vi "NPSV test.vi"() -> ()   [LabVIEW 2019]
uses:
  DataDef.ctl
  <vilib>/NI/Modbus Library/API/Modbus API.lvclass
  <vilib>/WPC Systems Ltd/GECO Driver/Lib/GECOBase/GECO_Driver Class/GECO_Driver.lvclass
  <vilib>/WPC Systems Ltd/GECO Driver/Lib/GECOMotion/GECOMotion/_typedefine/Axis Select.ctl
  <vilib>/WPC Systems Ltd/GECO Driver/Lib/GECOBase/GECO_Driver Class/Motion/_typedefine/GECO_Stepper Output Configuration.ctl
  <vilib>/WPC Systems Ltd/GECO Driver/Lib/GECOBase/GECO_Driver Class/Motion/_typedefine/GECO_Motion Operation Mode.ctl
  <vilib>/WPC Systems Ltd/GECO Driver/Lib/GECOBase/GECO_Driver Class/GECO_SlotName.ctl
  <vilib>/WPC Systems Ltd/GECO Driver/Lib/GECOBase/GECO_Driver Class/Motion/_typedefine/GECO_ActiveHighLow.ctl
  <vilib>/WPC Systems Ltd/GECO Driver/Lib/GECOMotion/GECOMotion/GECO Motion.lvclass
  GyroDef.ctl
  <vilib>/Platform/TimedLoop/XDataNode/timing_clust.ctl
  <vilib>/Platform/TimedLoop/XDataNode/nitl_modes.ctl
  <vilib>/Platform/TimedLoop/XDataNode/wakeup.ctl
  <vilib>/NI/Modbus Library/API/Slave/Modbus Slave.lvclass
  C:/Program Files (x86)/National Instruments/LabVIEW 2019/vi.lib/NI/Modbus Library/API/Modbus API.lvclass
  <vilib>/addons/control/pid/pid.llb/PID (DBL).vi
  <vilib>/NI/Modbus Library/API/Wrapper/Create TCP Slave.vi
  <vilib>/WPC Systems Ltd/GECO Driver/GECODriver/GECO_Initialize_RT/Initialize VIs/Initialize_GECOUnoRT_4HX.vi
  <vilib>/platform/TimedLoop/XDataNode/XDataNode.xnode
  <vilib>/addons/control/pid/NI_PID_pid.lvlib
  <vilib>/NI/Modbus Library/API/Wrapper/API Main.lvlib
  <vilib>/Platform/TimedLoop/XDataNode/XDNodeRunTimeDep.lvlib
panel:
  out "error out":errorcluster
  out "Axis 1":T1
  out "Axis 2":T1
  out "Axis 3":T1
  out "Program Period":u32
  in  "Main Setting Tab":T2(tab)
  in  "PID gains setting Tab":enum32{"Axis 1", "Axis 2", "Axis 3"}(tab)
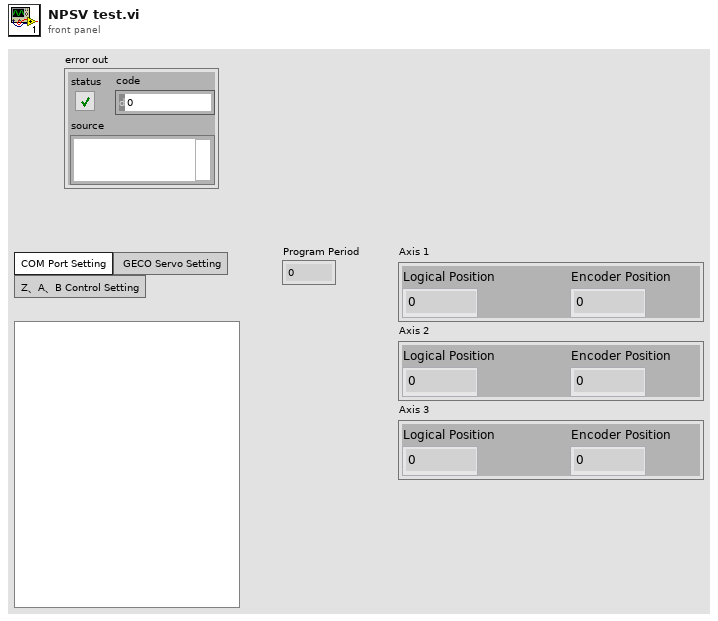
[diagram p1: front panel]
types:
  T1 = cluster{"Encoder Position":i32, "Logical Position":i32}
  T2 = enum32{"COM Port Setting", " GECO Servo Setting", "Z、A、B Control Setting"}
  T3 = typedef "DataDef.ctl" = cluster{"address starting":u16, "狀態":enum16{"初始化", "讀取", "寫入", "停止"}, "理想角度":cluster{"A":dbl, "B":dbl}, "register values":i16[], "Modbus COM":refnum<class "Modbus API.lvclass">, "TCP slave port":u16, " baud rate":u32, "Byte bits":u16, "ServoButtonControl":cluster{"三軸同退":bool, "三軸同進":bool, "三軸後退":bool, "三軸前進":bool, "二軸後退":bool, "二軸前進":bool, "一軸後退":bool, "一軸前進":bool}, "Serial Number":string, "GECO_Driver out":refnum<class "GECO_Driver.lvclass">, "number of inputs":u16, "ServoSetting":cluster{"Axis Select":T4, "Stepper Output Configuration":T5, "Motion Operation Mode":T6, "Motion Controller Slot":T7, "Singel Axis Move Paramters":cluster{"Motion Operation Mode":T6, "Target Position (0)":i32, "Velocity (10000)":i32, "Acceleration (100000)":u32, "Deacceleration (100000)":u32}, "Reverse":cluster{"Reverse Enable":bool, "Reverse Polarity":T8}, "Forward":cluster{"Forward Enable":bool, "Forward Polarity":T8}}, "GECO Motion out":refnum<class "GECO Motion.lvclass">, "Servo on":bool, "Axis 1 Position":cluster{"Encoder Position":i32, "Logical Position":i32}, "Axis 2 Position":cluster{"Encoder Position":i32, "Logical Position":i32}, "Axis 3 Position":cluster{"Encoder Position":i32, "Logical Position":i32}, "PIDSetting":cluster{"Z":i32, "A":i32, "B":i32, "Move Setting":T9, "Axis Pulse":dbl, "Axis Length":dbl, "PID gains ":cluster{"proportional gain (Kc)":dbl, "integral time (Ti, min)":dbl, "derivative time (Td, min)":dbl}}, "resource name":tag, "Save Path":refnum<file>}
  T4 = typedef "GECO Motion.lvclass/Axis Select.ctl" = enum16{"Axis 1", "Axis 2", "Axis 3", "Axis 4"}
  T5 = typedef "GECO_Driver.lvclass/GECO_Stepper Output Configuration.ctl" = enum16{"Step/Dir(One Pulse)", "CW/CCW(Two Pulse)"}
  T6 = typedef "GECO_Driver.lvclass/GECO_Motion Operation Mode.ctl" = enum16{"Absolute Position", "Relative Position", "Velocity"}
  T7 = typedef "GECO_Driver.lvclass/GECO_SlotName.ctl" = enum16{"C1", "C2", "C3", "C4"}
  T8 = typedef "GECO_Driver.lvclass/GECO_ActiveHighLow.ctl" = enum16{"Active High", "Active Low"}
  T9 = typedef "­y¸ñ.ctl" = u16
  T10 = typedef "GyroDef.ctl" = cluster{"Byte bits":u16, "baud rate":u32, "實際角度":cluster{"A":dbl, "B":dbl}, "COM Port":refnum<visa-resource-name>, "Save Path":refnum<file>}
  T11 = typedef "XDNodeRunTimeDep.lvlib/timing_clust.ctl" = cluster{"Expected End [f-1]":u64, "Actual End [f-1]":u64, "Finished Late? [f-1]":bool, "Expected End [i-1]":u64, "Actual End [i-1]":u64, "Finished Late? [i-1]":bool, "Expected Start [i]":u64, "Actual Start [i]":u64, "Expected Start [f]":u64, "Actual Start [f]":u64, "Source Name":string, "Structure Name":string, "Period":i64, "Deadline":i64, "Offset":i64, "Start":i64, "Priority":i32, "Timeout":i32, "Mode":T12, "Wakeup Reason":T13, "Error":errorcluster, "Source Type":string, "Secondary Source Type":string, "Global End Time":u64, "Global Start Time":u64, "Frame Duration":u64, "Iteration Duration":u64, "Assigned CPU":i32, "I/O Scan Engine Mode":u32}
  T12 = typedef "XDNodeRunTimeDep.lvlib/nitl_modes.ctl" = enum32{"No Change", "Process missed periods, maintain original phase", "Discard missed periods, maintain original phase", "Process missed periods, ignore original phase", "Discard missed periods, ignore original phase"}
  T13 = typedef "XDNodeRunTimeDep.lvlib/wakeup.ctl" = enum32{"Normal", "Aborted", "Asynchronous wakeup", "Timing source error", "Timed loop error", "Timeout"}
  T14 = cluster{"Motion Operation Mode":T6, "Target Position (0)":i32, "Velocity (10000)":i32, "Acceleration (100000)":u32, "Deacceleration (100000)":u32}
  T15 = cluster{"Forward Enable":bool, "Forward Polarity":T8}
  T16 = cluster{"Reverse Enable":bool, "Reverse Polarity":T8}
  T17 = cluster{"三軸同退":bool, "三軸同進":bool, "三軸後退":bool, "三軸前進":bool, "二軸後退":bool, "二軸前進":bool, "一軸後退":bool, "一軸前進":bool, "Reset Encoder Position":bool, "AlarmReset":bool}[]
  T18 = cluster{"三軸同退":bool, "三軸同進":bool, "三軸後退":bool, "三軸前進":bool, "二軸後退":bool, "二軸前進":bool, "一軸後退":bool, "一軸前進":bool, "Reset Encoder Position":bool, "AlarmReset":bool}
  T19 = enum16{"open", "replace", "create", "open or create", "replace or create", "replace or create with confirmation"}
  T20 = cluster{"Logical Position":i32, "Encoder Position":i32}
  T21 = enum16{"Step/Dir(One Pulse)", "CW/CCW(Two Pulse)"}
  T22 = enum16{"Absolute Position", "Relative Position", "Velocity"}
  T23 = cluster{"proportional gain (Kc)":dbl, "integral time (Ti, min)":dbl, "derivative time (Td, min)":dbl}
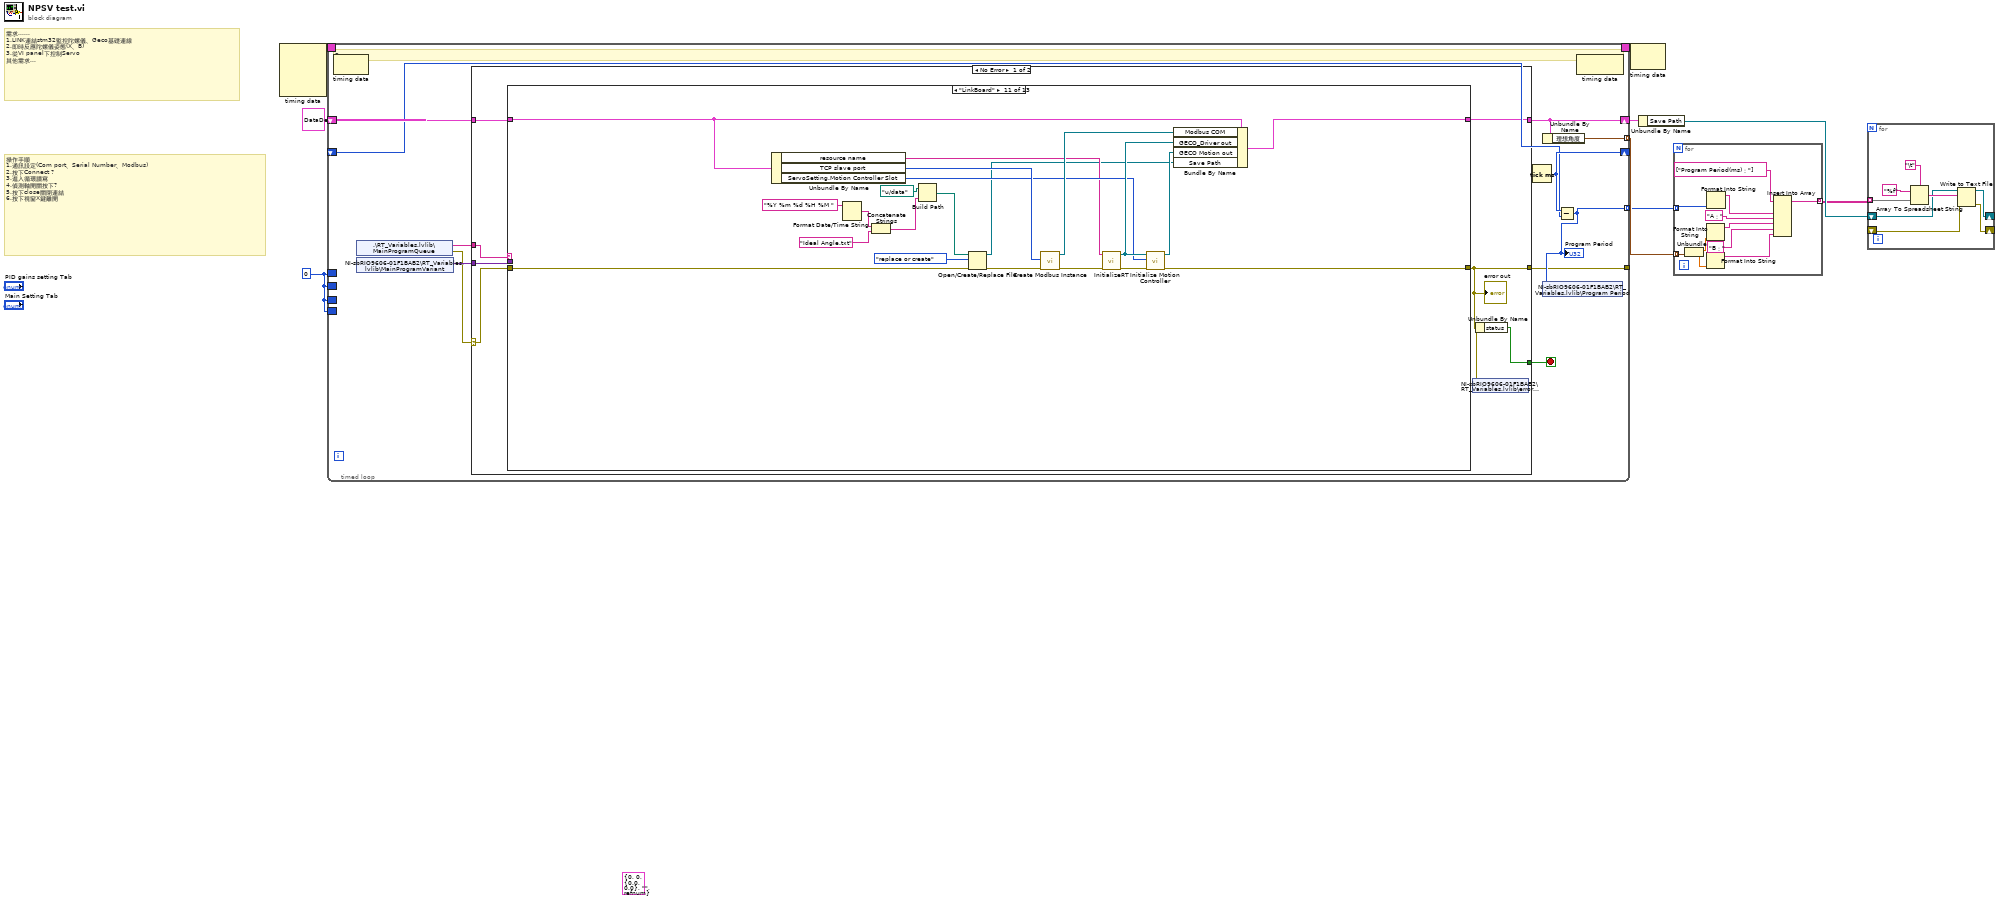
[diagram p0: block diagram]
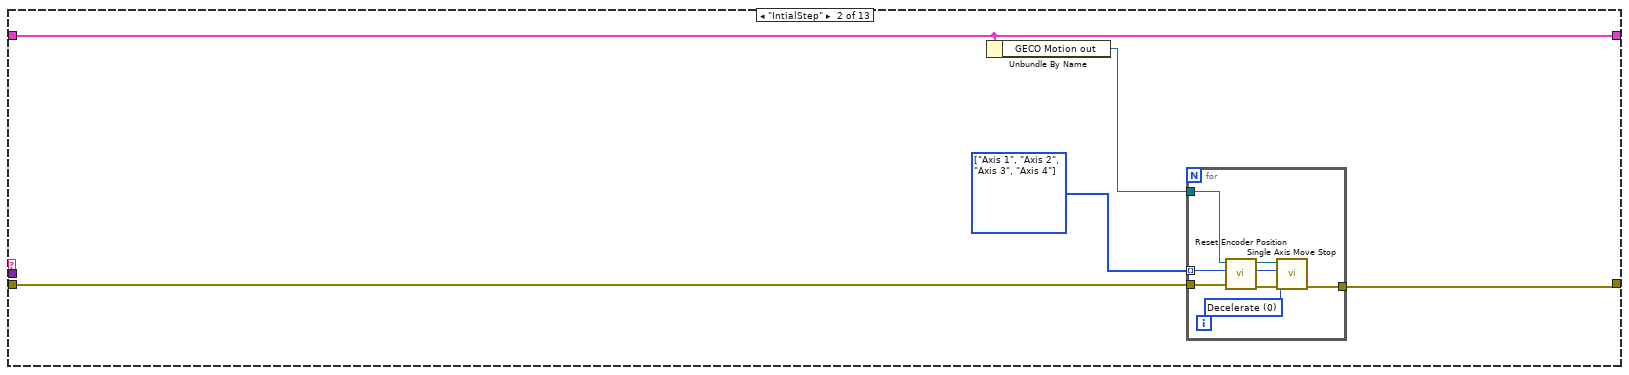
[diagram p3: hidden frame]
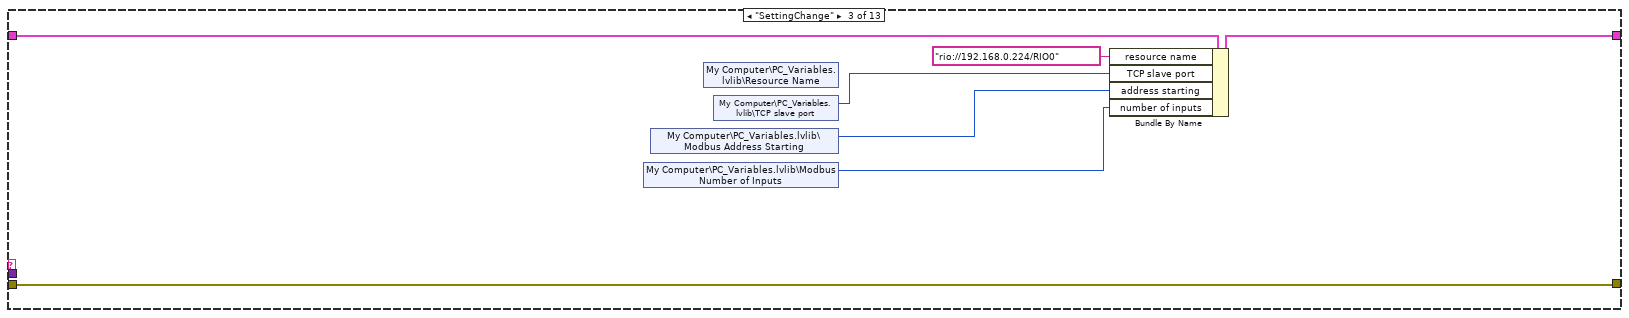
[diagram p4: hidden frame]
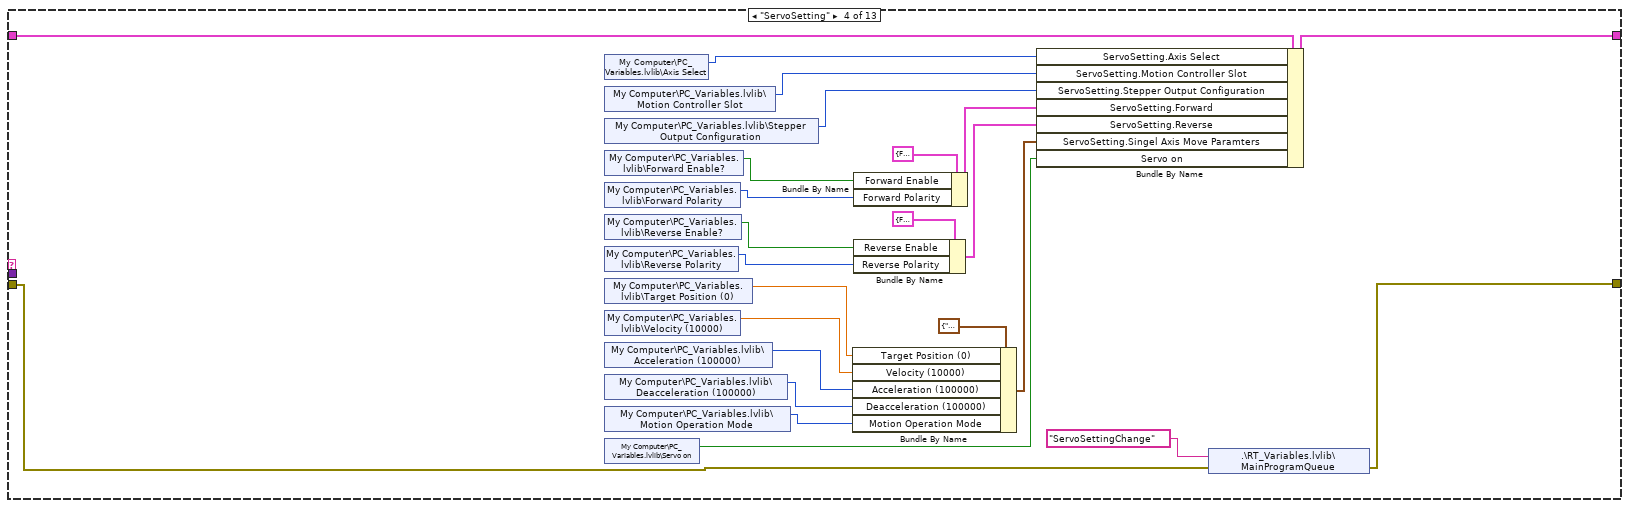
[diagram p5: hidden frame]
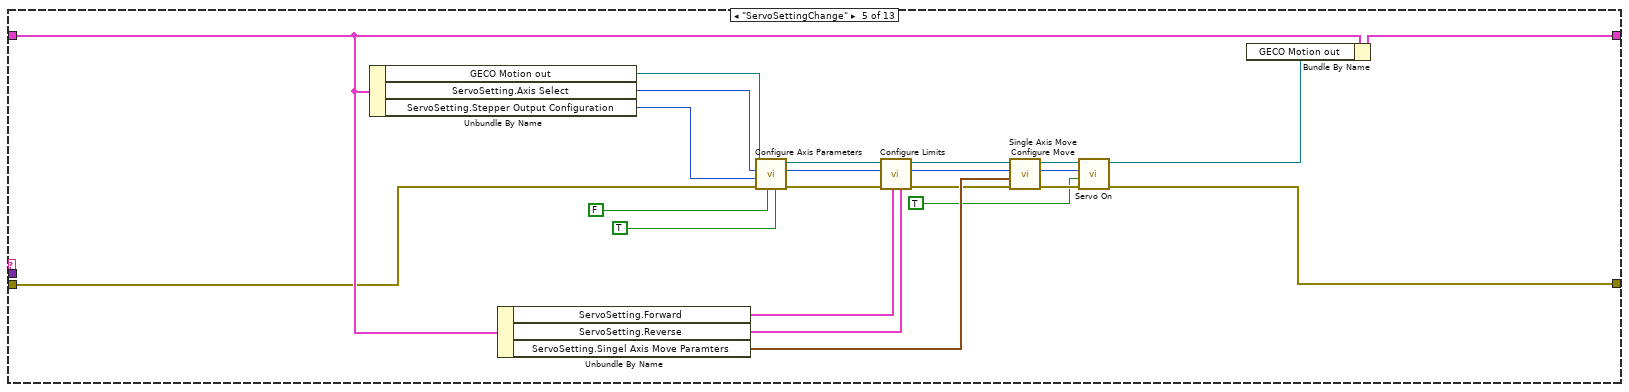
[diagram p6: hidden frame]
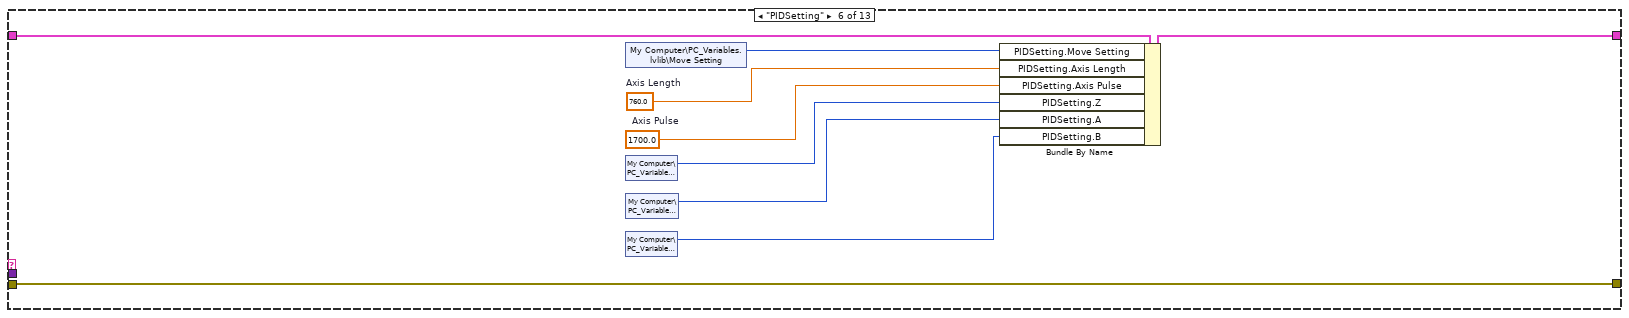
[diagram p7: hidden frame]
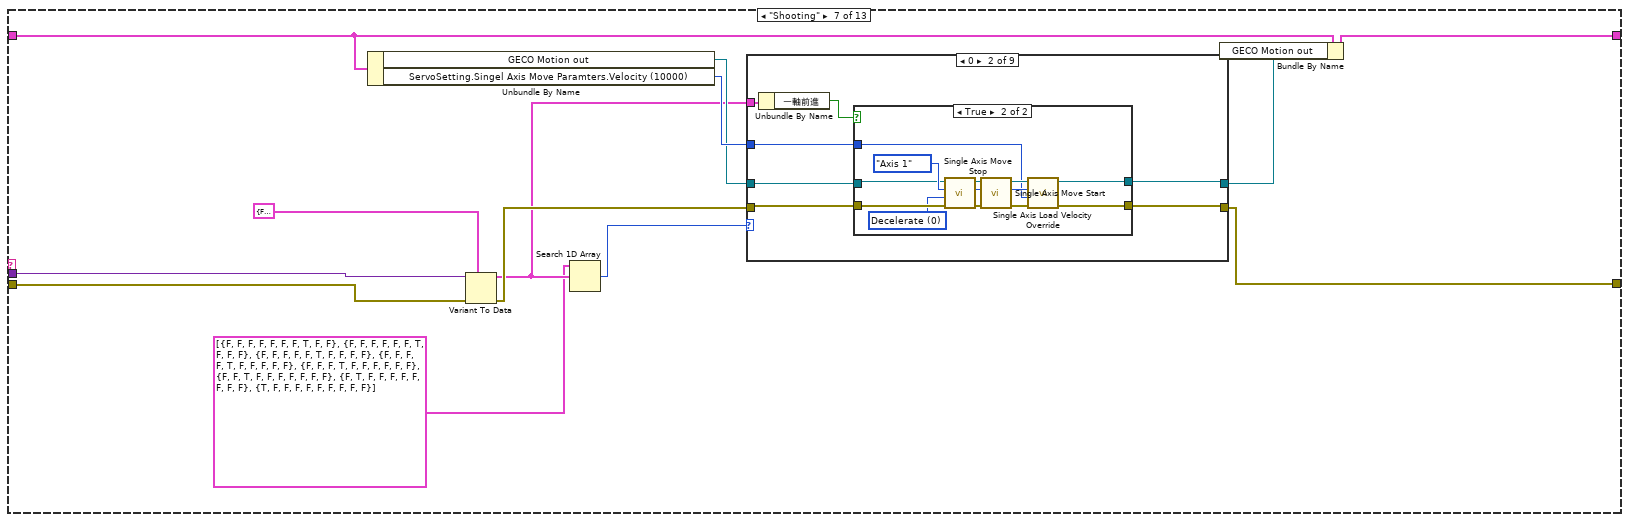
[diagram p8: hidden frame]
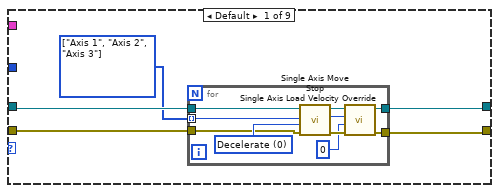
[diagram p9: hidden frame]
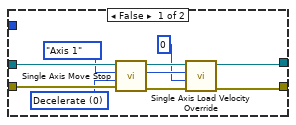
[diagram p10: hidden frame]
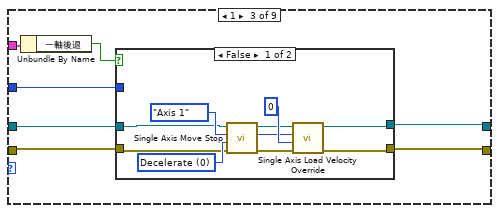
[diagram p11: hidden frame]
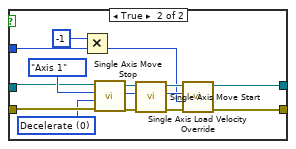
[diagram p12: hidden frame]
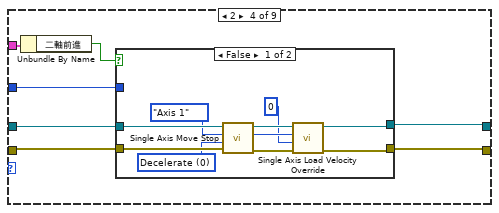
[diagram p13: hidden frame]
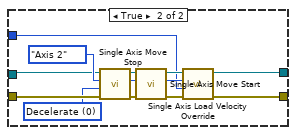
[diagram p14: hidden frame]
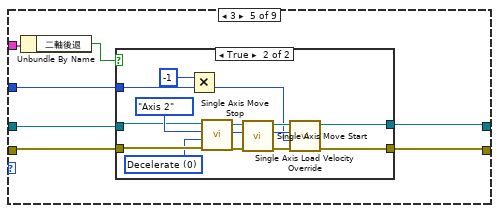
[diagram p15: hidden frame]
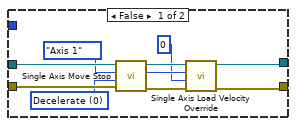
[diagram p16: hidden frame]
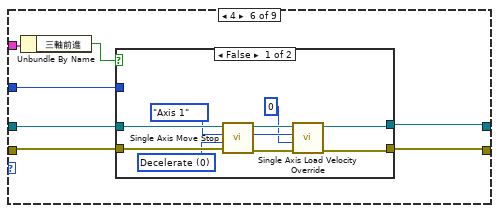
[diagram p17: hidden frame]
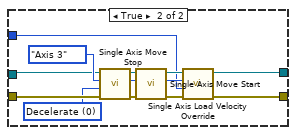
[diagram p18: hidden frame]
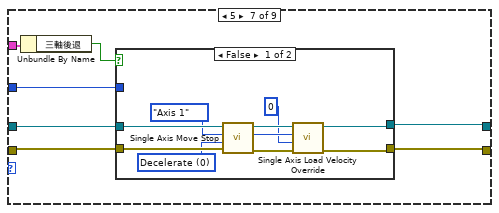
[diagram p19: hidden frame]
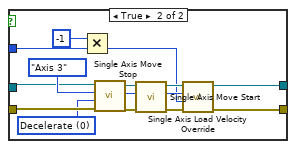
[diagram p20: hidden frame]
diagram:
  w8 = 0
  (unwired) T10 {"Byte bits"=0, "baud rate"=0, "實際角度"={"A"=0.0, "B"=0.0}, "COM Port"="", "Save Path"=refnum}
  # "操作手順\n1.通訊設定(Com port、Serial Number、Modbus)\n2.按下Connect ?\n3.進入循環讀寫\n4.偵測軸開關按下?\n5.按下close關閉連結\n6.按下視窗X鍵離開"
  # "需求......\n1.LINK連結stm32監控陀螺儀、Geco基礎連線\n2.即時反應陀螺儀姿態(X、B)\n3.從VI panel下控制Servo\n其他需求..."
  n1 = node-c288() -> (w2:T11)  [unwired: 4 in]
  n2 = timed-loop {
    shift-right: [w16] -> w5
    shift-left: T3 {"address starting"=0, "狀態"=enum."初始化", "理想角度"={"A"=0.0, "B"=0.0}, "register values"=[], "Modbus COM"=refnum, "TCP slave port"=1, " baud rate"=0, "Byte bits"=0, "ServoButtonControl"={"三軸同退"=FALSE, "三軸同進"=FALSE, "三軸後退"=FALSE, "三軸前進"=FALSE, "二軸後退"=FALSE, "二軸前進"=FALSE, "一軸後退"=FALSE, "一軸前進"=FALSE}, "Serial Number"="", "GECO_Driver out"=refnum, "number of inputs"=0, "ServoSetting"={"Axis Select"=enum."Axis 1", "Stepper Output Configuration"=enum."Step/Dir(One Pulse)", "Motion Operation Mode"=enum."Absolute Position", "Motion Controller Slot"=enum."C1", "Singel Axis Move Paramters"={"Motion Operation Mode"=enum."Velocity", "Target Position (0)"=10000, "Velocity (10000)"=1, "Acceleration (100000)"=100000, "Deacceleration (100000)"=1}, "Reverse"={"Reverse Enable"=FALSE, "Reverse Polarity"=enum."Active Low"}, "Forward"={"Forward Enable"=FALSE, "Forward Polarity"=enum."Active Low"}}, "GECO Motion out"=refnum, "Servo on"=FALSE, "Axis 1 Position"={"Encoder Position"=0, "Logical Position"=0}, "Axis 2 Position"={"Encoder Position"=0, "Logical Position"=0}, "Axis 3 Position"={"Encoder Position"=0, "Logical Position"=0}, "PIDSetting"={"Z"=10000, "A"=10000, "B"=10000, "Move Setting"=1, "Axis Pulse"=10000.0, "Axis Length"=10000.0, "PID gains "={"proportional gain (Kc)"=1.0, "integral time (Ti, min)"=0.01, "derivative time (Td, min)"=0.0}}, "resource name"="", "Save Path"=refnum} -> [w19]
    shift-right: [w18] -> _
    shift-left: _ -> [w17]
    border: w8 -> [_]
    border: w8 -> [_]
    border: w8 -> [_]
    border: w8 -> [_]
    tunnel: [w15] -> w7 mode=indexing
    tunnel: [w14] -> w6 mode=indexing
    tunnel: [w13] -> _
    timing: w2 -> [_]
    timing-out: [_] -> w1
    stop <- w20 stop-if-true
    # "Process"
    n3 = node-c288() -> ()  [unwired: 1 in, 1 out]
    n4 = shared-variable ".\\RT_Variables.lvlib\\MainProgramQueue"() -> (w11:string, error out=w10:errorcluster)  [unwired: 1 in]
    n5 = shared-variable "NI-sbRIO9606-01F1BAB2\\RT_Variables.lvlib\\MainProgramVariant"() -> (w12:variant)  [unwired: 1 in, 1 out]
    n6 = case shown="No Error" w10 {
      selector: w10 -> [w27 w633]
      tunnel: [w26 TRUE] -> w20
      tunnel: [w29 w634] -> w16
      tunnel: w19 -> [w28 w634]
      tunnel: [w25 w633] -> w13
      tunnel: w12 -> [w24 _]
      tunnel: w11 -> [w23 _]
      frame No Error {
        n7 = case shown="\"LinkBoard\"" w23 {
          tunnel: [w31 w33 w50 w74 w98 w106 w118 w408 w542 w558 w591 w613 w624] -> w29
          tunnel: w28 -> [w31 w33 w51 w75 w97 w107 w112 w410 w545 w561 w592 w615 w624]
          tunnel: w27 -> [w30 w32 w47 w53 w90 w99 w120 w401 w544 w560 w574 w617 w622]
          tunnel: [w30 w36 w47 w54 w84 w99 w111 w409 w540 w556 w586 w616 w623] -> w25
          tunnel: w24 -> [_ _ _ _ _ _ w119 _ _ _ _ _ _]
          frame Default {
          }
          frame "IntialStep" {
            w34 = T4[] [enum."Axis 1", enum."Axis 2", enum."Axis 3", enum."Axis 4"] items=["Axis 1", "Axis 2", "Axis 3", "Axis 4"]
            n8 = Unbundle By Name(w33) -> ("GECO Motion out"=w35:refnum<class "GECO Motion.lvclass">)
            n9 = for {
              tunnel: [w39] -> w36
              tunnel: w35 -> [w44]
              tunnel: w34 -> [w43] mode=indexing
              tunnel: w32 -> [w37]
              w38 = u16 0 items=["Decelerate", "Halt"] ("Motion Stop Type")
              n10 = call <vilib>:"Reset Encoder Position.vi"("error in (no error)"=w37, "Axis Select"=w43, "GECO Motion in"=w44) -> ("error out"=w42:errorcluster, "Axis Select out"=w41:T4, "GECO Motion out"=w40:refnum<class "GECO Motion.lvclass">)  [unwired: 6 in]
              n11 = call <vilib>:"Single Axis Move Stop.vi"("error in (no error)"=w42, "Motion Stop Type"=w38, "Axis Select"=w41, "GECO Motion in"=w40) -> ("error out"=w39:errorcluster)  [unwired: 5 in, 2 out]
            }
          }
          frame "SettingChange" {
            n12 = shared-variable "My Computer\\PC_Variables.lvlib\\Modbus Number of Inputs"() -> (w46:u32)  [unwired: 1 in, 1 out]
            n13 = shared-variable "My Computer\\PC_Variables.lvlib\\Modbus Address Starting"() -> (w48:u32)  [unwired: 1 in, 1 out]
            n14 = shared-variable "My Computer\\PC_Variables.lvlib\\Resource Name"() -> ()  [unwired: 1 in, 2 out]
            n15 = shared-variable "My Computer\\PC_Variables.lvlib\\TCP slave port"() -> (w49:u32)  [unwired: 1 in, 1 out]
            n16 = Bundle By Name(cluster=w51, "resource name"=tag "rio://192.168.0.224/RIO0", "TCP slave port"=w49, "address starting"=w48, "number of inputs"=w46) -> (w50:T3)
          }
          frame "ServoSetting" {
            n17 = shared-variable "My Computer\\PC_Variables.lvlib\\Axis Select"() -> (w73:enum16{"Axis 1", "Axis 2", "Axis 3", "Axis 4"})  [unwired: 1 in, 1 out]
            n18 = shared-variable "My Computer\\PC_Variables.lvlib\\Motion Controller Slot"() -> (w72:enum16{"C1", "C2", "C3", "C4"})  [unwired: 1 in, 1 out]
            n19 = shared-variable "My Computer\\PC_Variables.lvlib\\Stepper Output Configuration"() -> (w71:T21)  [unwired: 1 in, 1 out]
            n20 = shared-variable "My Computer\\PC_Variables.lvlib\\Forward Enable?"() -> (w59:bool)  [unwired: 1 in, 1 out]
            n21 = shared-variable "My Computer\\PC_Variables.lvlib\\Forward Polarity"() -> (w60:enum16{"Active High", "Active Low"})  [unwired: 1 in, 1 out]
            n22 = shared-variable "My Computer\\PC_Variables.lvlib\\Reverse Enable?"() -> (w62:bool)  [unwired: 1 in, 1 out]
            n23 = shared-variable "My Computer\\PC_Variables.lvlib\\Reverse Polarity"() -> (w61:enum16{"Active High", "Active Low"})  [unwired: 1 in, 1 out]
            n24 = shared-variable "My Computer\\PC_Variables.lvlib\\Target Position (0)"() -> (w63:dbl)  [unwired: 1 in, 1 out]
            n25 = shared-variable "My Computer\\PC_Variables.lvlib\\Velocity (10000)"() -> (w64:dbl)  [unwired: 1 in, 1 out]
            n26 = shared-variable "My Computer\\PC_Variables.lvlib\\Acceleration (100000)"() -> (w65:u32)  [unwired: 1 in, 1 out]
            n27 = shared-variable "My Computer\\PC_Variables.lvlib\\Deacceleration (100000)"() -> (w66:u32)  [unwired: 1 in, 1 out]
            n28 = shared-variable "My Computer\\PC_Variables.lvlib\\Motion Operation Mode"() -> (w67:T22)  [unwired: 1 in, 1 out]
            n29 = shared-variable "My Computer\\PC_Variables.lvlib\\Servo on"() -> (w55:bool)  [unwired: 1 in, 1 out]
            n30 = Bundle By Name(cluster=T14 {"Motion Operation Mode"=enum."Absolute Position", "Target Position (0)"=0, "Velocity (10000)"=10000, "Acceleration (100000)"=100000, "Deacceleration (100000)"=100000} ("Singel Axis Move Paramters"), "Target Position (0)"=w63, "Velocity (10000)"=w64, "Acceleration (100000)"=w65, "Deacceleration (100000)"=w66, "Motion Operation Mode"=w67) -> (w56:T14)
            n31 = Bundle By Name(cluster=T15 {"Forward Enable"=FALSE, "Forward Polarity"=enum."Active Low"} ("Forward"), "Forward Enable"=w59, "Forward Polarity"=w60) -> (w58:T15)
            n32 = Bundle By Name(cluster=T16 {"Reverse Enable"=FALSE, "Reverse Polarity"=enum."Active Low"} ("Reverse"), "Reverse Enable"=w62, "Reverse Polarity"=w61) -> (w57:T16)
            n33 = Bundle By Name(cluster=w75, "ServoSetting.Axis Select"=w73, "ServoSetting.Motion Controller Slot"=w72, "ServoSetting.Stepper Output Configuration"=w71, "ServoSetting.Forward"=w58, "ServoSetting.Reverse"=w57, "ServoSetting.Singel Axis Move Paramters"=w56, "Servo on"=w55) -> (w74:T3)
            n34 = shared-variable ".\\RT_Variables.lvlib\\MainProgramQueue"("ServoSettingChange", error in=w53) -> (error out=w54:errorcluster)
          }
          frame "ServoSettingChange" {
            n35 = Unbundle By Name(w97) -> ("GECO Motion out"=w91:refnum<class "GECO Motion.lvclass">, "ServoSetting.Axis Select"=w95:T4, "ServoSetting.Stepper Output Configuration"=w94:T5)
            n36 = Unbundle By Name(w97) -> ("ServoSetting.Forward"=w77:T15, "ServoSetting.Reverse"=w76:T16, "ServoSetting.Singel Axis Move Paramters"=w96:T14)
            n37 = call <vilib>:"Configure Axis Parameters.vi"("Reverse Encoder Direction?"=TRUE, "Reverse Axis Direction?"=FALSE, "error in (no error)"=w90, "Stepper Output Configuration"=w94, "Axis Select"=w95, "GECO Motion in"=w91) -> ("error out"=w81:errorcluster, "Axis Select out"=w83:T4, "GECO Motion out"=w82:refnum<class "GECO Motion.lvclass">)  [unwired: 3 in]
            n38 = call <vilib>:"Configure Limits.vi"("Reverse"=w76, "Forward"=w77, "error in (no error)"=w81, "Axis Select"=w83, "GECO Motion in"=w82) -> ("error out"=w78:errorcluster, "Axis Select out"=w79:T4, "GECO Motion out"=w80:refnum<class "GECO Motion.lvclass">)  [unwired: 4 in]
            n39 = call <vilib>:"Single Axis Move Configure Move.vi"("error in (no error)"=w78, "Singel Axis Move Paramters"=w96, "Axis Select"=w79, "GECO Motion in"=w80) -> ("error out"=w87:errorcluster, "Axis Select out"=w88:T4, "GECO Motion out"=w89:refnum<class "GECO Motion.lvclass">)  [unwired: 5 in]
            n40 = call <vilib>:"Servo On.vi"("error in (no error)"=w87, "Servo On"=TRUE, "Axis Select"=w88, "GECO Motion in"=w89) -> ("error out"=w84:errorcluster, "GECO Motion out"=w85:refnum<class "GECO Motion.lvclass">)  [unwired: 5 in, 1 out]
            n41 = Bundle By Name(cluster=w97, "GECO Motion out"=w85) -> (w98:T3)
          }
          frame "PIDSetting" {
            w103 = 1700.0  # Axis Pulse
            w104 = 760.0  # Axis Length
            n42 = shared-variable "My Computer\\PC_Variables.lvlib\\Move Setting"() -> (w105:u16)  [unwired: 1 in, 1 out]
            n43 = shared-variable "My Computer\\PC_Variables.lvlib\\Z"() -> (w102:i32)  [unwired: 1 in, 1 out]
            n44 = shared-variable "My Computer\\PC_Variables.lvlib\\A"() -> (w101:i32)  [unwired: 1 in, 1 out]
            n45 = shared-variable "My Computer\\PC_Variables.lvlib\\B"() -> (w100:i32)  [unwired: 1 in, 1 out]
            n46 = Bundle By Name(cluster=w107, "PIDSetting.Move Setting"=w105, "PIDSetting.Axis Length"=w104, "PIDSetting.Axis Pulse"=w103, "PIDSetting.Z"=w102, "PIDSetting.A"=w101, "PIDSetting.B"=w100) -> (w106:T3)
          }
          frame "Shooting" {
            n47 = Unbundle By Name(w112) -> ("GECO Motion out"=w114:refnum<class "GECO Motion.lvclass">, "ServoSetting.Singel Axis Move Paramters.Velocity (10000)"=w115:i32)
            n48 = Variant To Data(error in=w120, type=T18 {"三軸同退"=FALSE, "三軸同進"=FALSE, "三軸後退"=FALSE, "三軸前進"=FALSE, "二軸後退"=FALSE, "二軸前進"=FALSE, "一軸後退"=FALSE, "一軸前進"=FALSE, "Reset Encoder Position"=FALSE, "AlarmReset"=FALSE} ("ServoButtonControl"), Variant=w119) -> (data=w110:T18, error out=w116:errorcluster)
            n49 = Search 1D Array(1D array=T17 [{"三軸同退"=FALSE, "三軸同進"=FALSE, "三軸後退"=FALSE, "三軸前進"=FALSE, "二軸後退"=FALSE, "二軸前進"=FALSE, "一軸後退"=FALSE, "一軸前進"=TRUE, "Reset Encoder Position"=FALSE, "AlarmReset"=FALSE}, {"三軸同退"=FALSE, "三軸同進"=FALSE, "三軸後退"=FALSE, "三軸前進"=FALSE, "二軸後退"=FALSE, "二軸前進"=FALSE, "一軸後退"=TRUE, "一軸前進"=FALSE, "Reset Encoder Position"=FALSE, "AlarmReset"=FALSE}, {"三軸同退"=FALSE, "三軸同進"=FALSE, "三軸後退"=FALSE, "三軸前進"=FALSE, "二軸後退"=FALSE, "二軸前進"=TRUE, "一軸後退"=FALSE, "一軸前進"=FALSE, "Reset Encoder Position"=FALSE, "AlarmReset"=FALSE}, {"三軸同退"=FALSE, "三軸同進"=FALSE, "三軸後退"=FALSE, "三軸前進"=FALSE, "二軸後退"=TRUE, "二軸前進"=FALSE, "一軸後退"=FALSE, "一軸前進"=FALSE, "Reset Encoder Position"=FALSE, "AlarmReset"=FALSE}, {"三軸同退"=FALSE, "三軸同進"=FALSE, "三軸後退"=FALSE, "三軸前進"=TRUE, "二軸後退"=FALSE, "二軸前進"=FALSE, "一軸後退"=FALSE, "一軸前進"=FALSE, "Reset Encoder Position"=FALSE, "AlarmReset"=FALSE}, {"三軸同退"=FALSE, "三軸同進"=FALSE, "三軸後退"=TRUE, "三軸前進"=FALSE, "二軸後退"=FALSE, "二軸前進"=FALSE, "一軸後退"=FALSE, "一軸前進"=FALSE, "Reset Encoder Position"=FALSE, "AlarmReset"=FALSE}, {"三軸同退"=FALSE, "三軸同進"=TRUE, "三軸後退"=FALSE, "三軸前進"=FALSE, "二軸後退"=FALSE, "二軸前進"=FALSE, "一軸後退"=FALSE, "一軸前進"=FALSE, "Reset Encoder Position"=FALSE, "AlarmReset"=FALSE}, {"三軸同退"=TRUE, "三軸同進"=FALSE, "三軸後退"=FALSE, "三軸前進"=FALSE, "二軸後退"=FALSE, "二軸前進"=FALSE, "一軸後退"=FALSE, "一軸前進"=FALSE, "Reset Encoder Position"=FALSE, "AlarmReset"=FALSE}], element=w110) -> (index of element=w117:i32)  [unwired: 1 in]
            n50 = case shown="0" w117 {
              tunnel: w116 -> [w124 w141 w171 w203 w233 w265 w295 w327 w364]
              tunnel: w115 -> [_ w140 w170 w202 w232 w264 w294 w326 w363]
              tunnel: w114 -> [w125 w142 w172 w204 w234 w266 w296 w328 w365]
              tunnel: [w122 w139 w169 w201 w231 w263 w293 w325 w362] -> w113
              tunnel: [w121 w138 w168 w200 w230 w262 w292 w324 w361] -> w111
              tunnel: w110 -> [_ w137 w167 w199 w229 w261 w291 w323 w360]
              frame Default {
                w123 = T4[] [enum."Axis 1", enum."Axis 2", enum."Axis 3"] items=["Axis 1", "Axis 2", "Axis 3", "Axis 4"] ("Start Axes Select")
                n51 = for {
                  tunnel: w124 -> [w134]
                  tunnel: w125 -> [w133]
                  tunnel: w123 -> [w132] mode=indexing
                  tunnel: [w127] -> w122
                  tunnel: [w128] -> w121
                  w135 = u16 0 items=["Decelerate", "Halt"] ("Motion Stop Type")
                  n52 = call <vilib>:"Single Axis Move Stop.vi"("error in (no error)"=w134, "Motion Stop Type"=w135, "Axis Select"=w132, "GECO Motion in"=w133) -> ("error out"=w130:errorcluster, "Axis Select out"=w129:T4, "GECO Motion out"=w131:refnum<class "GECO Motion.lvclass">)  [unwired: 5 in]
                  n53 = call <vilib>:"Single Axis Load Velocity Override.vi"("error in (no error)"=w130, "Override Velosity Value"=0, "Axis Select"=w129, "GECO Motion in"=w131) -> ("error out"=w128:errorcluster, "GECO Motion out"=w127:refnum<class "GECO Motion.lvclass">)  [unwired: 5 in, 1 out]
                }
              }
              frame 0 {
                n54 = Unbundle By Name(w137) -> ("一軸前進"=w136:bool)
                n55 = case shown="True" w136 {
                  tunnel: w142 -> [w152 w158]
                  tunnel: w141 -> [w151 w157]
                  tunnel: w140 -> [_ w162]
                  tunnel: [w143 w161] -> w139
                  tunnel: [w144 w160] -> w138
                  frame False {
                    w150 = u16 0 items=["Decelerate", "Halt"] ("Motion Stop Type")
                    n56 = call <vilib>:"Single Axis Move Stop.vi"("error in (no error)"=w151, "Motion Stop Type"=w150, "Axis Select"=Axis_Select."Axis 1", "GECO Motion in"=w152) -> ("error out"=w147:errorcluster, "Axis Select out"=w146:T4, "GECO Motion out"=w148:refnum<class "GECO Motion.lvclass">)  [unwired: 5 in]
                    n57 = call <vilib>:"Single Axis Load Velocity Override.vi"("error in (no error)"=w147, "Override Velosity Value"=0, "Axis Select"=w146, "GECO Motion in"=w148) -> ("error out"=w144:errorcluster, "GECO Motion out"=w143:refnum<class "GECO Motion.lvclass">)  [unwired: 5 in, 1 out]
                  }
                  frame True {
                    w156 = u16 0 items=["Decelerate", "Halt"] ("Motion Stop Type")
                    n58 = call <vilib>:"Single Axis Move Stop.vi"("error in (no error)"=w157, "Motion Stop Type"=w156, "Axis Select"=Axis_Select."Axis 1", "GECO Motion in"=w158) -> ("error out"=w154:errorcluster, "Axis Select out"=w153:T4, "GECO Motion out"=w155:refnum<class "GECO Motion.lvclass">)  [unwired: 5 in]
                    n59 = call <vilib>:"Single Axis Move Start.vi"("error in (no error)"=w154, "Axis Select"=w153, "GECO Motion in"=w155) -> ("error out"=w164:errorcluster, "Axis Select out"=w163:T4, "GECO Motion out"=w165:refnum<class "GECO Motion.lvclass">)  [unwired: 6 in]
                    n60 = call <vilib>:"Single Axis Load Velocity Override.vi"("error in (no error)"=w164, "Override Velosity Value"=w162, "Axis Select"=w163, "GECO Motion in"=w165) -> ("error out"=w160:errorcluster, "GECO Motion out"=w161:refnum<class "GECO Motion.lvclass">)  [unwired: 5 in, 1 out]
                  }
                }
              }
              frame 1 {
                n61 = Unbundle By Name(w167) -> ("一軸後退"=w166:bool)
                n62 = case shown="False" w166 {
                  tunnel: w172 -> [w178 w186]
                  tunnel: w171 -> [w176 w185]
                  tunnel: w170 -> [_ w194]
                  tunnel: [w180 w193] -> w169
                  tunnel: [w181 w192] -> w168
                  frame False {
                    w177 = u16 0 items=["Decelerate", "Halt"] ("Motion Stop Type")
                    n63 = call <vilib>:"Single Axis Move Stop.vi"("error in (no error)"=w176, "Motion Stop Type"=w177, "Axis Select"=Axis_Select."Axis 1", "GECO Motion in"=w178) -> ("error out"=w174:errorcluster, "Axis Select out"=w173:T4, "GECO Motion out"=w175:refnum<class "GECO Motion.lvclass">)  [unwired: 5 in]
                    n64 = call <vilib>:"Single Axis Load Velocity Override.vi"("error in (no error)"=w174, "Override Velosity Value"=0, "Axis Select"=w173, "GECO Motion in"=w175) -> ("error out"=w181:errorcluster, "GECO Motion out"=w180:refnum<class "GECO Motion.lvclass">)  [unwired: 5 in, 1 out]
                  }
                  frame True {
                    w184 = u16 0 items=["Decelerate", "Halt"] ("Motion Stop Type")
                    n65 = Multiply(x=-1, y=w194) -> (x*y=w191:i32)
                    n66 = call <vilib>:"Single Axis Move Stop.vi"("error in (no error)"=w185, "Motion Stop Type"=w184, "Axis Select"=Axis_Select."Axis 1", "GECO Motion in"=w186) -> ("error out"=w188:errorcluster, "Axis Select out"=w183:T4, "GECO Motion out"=w189:refnum<class "GECO Motion.lvclass">)  [unwired: 5 in]
                    n67 = call <vilib>:"Single Axis Move Start.vi"("error in (no error)"=w188, "Axis Select"=w183, "GECO Motion in"=w189) -> ("error out"=w196:errorcluster, "Axis Select out"=w195:T4, "GECO Motion out"=w197:refnum<class "GECO Motion.lvclass">)  [unwired: 6 in]
                    n68 = call <vilib>:"Single Axis Load Velocity Override.vi"("error in (no error)"=w196, "Override Velosity Value"=w191, "Axis Select"=w195, "GECO Motion in"=w197) -> ("error out"=w192:errorcluster, "GECO Motion out"=w193:refnum<class "GECO Motion.lvclass">)  [unwired: 5 in, 1 out]
                  }
                }
              }
              frame 2 {
                n69 = Unbundle By Name(w199) -> ("二軸前進"=w198:bool)
                n70 = case shown="False" w198 {
                  tunnel: w204 -> [w214 w220]
                  tunnel: w203 -> [w213 w219]
                  tunnel: w202 -> [_ w224]
                  tunnel: [w205 w223] -> w201
                  tunnel: [w206 w222] -> w200
                  frame False {
                    w212 = u16 0 items=["Decelerate", "Halt"] ("Motion Stop Type")
                    n71 = call <vilib>:"Single Axis Move Stop.vi"("error in (no error)"=w213, "Motion Stop Type"=w212, "Axis Select"=Axis_Select."Axis 1", "GECO Motion in"=w214) -> ("error out"=w209:errorcluster, "Axis Select out"=w208:T4, "GECO Motion out"=w210:refnum<class "GECO Motion.lvclass">)  [unwired: 5 in]
                    n72 = call <vilib>:"Single Axis Load Velocity Override.vi"("error in (no error)"=w209, "Override Velosity Value"=0, "Axis Select"=w208, "GECO Motion in"=w210) -> ("error out"=w206:errorcluster, "GECO Motion out"=w205:refnum<class "GECO Motion.lvclass">)  [unwired: 5 in, 1 out]
                  }
                  frame True {
                    w218 = u16 0 items=["Decelerate", "Halt"] ("Motion Stop Type")
                    n73 = call <vilib>:"Single Axis Move Stop.vi"("error in (no error)"=w219, "Motion Stop Type"=w218, "Axis Select"=Axis_Select."Axis 2", "GECO Motion in"=w220) -> ("error out"=w216:errorcluster, "Axis Select out"=w215:T4, "GECO Motion out"=w217:refnum<class "GECO Motion.lvclass">)  [unwired: 5 in]
                    n74 = call <vilib>:"Single Axis Move Start.vi"("error in (no error)"=w216, "Axis Select"=w215, "GECO Motion in"=w217) -> ("error out"=w226:errorcluster, "Axis Select out"=w225:T4, "GECO Motion out"=w227:refnum<class "GECO Motion.lvclass">)  [unwired: 6 in]
                    n75 = call <vilib>:"Single Axis Load Velocity Override.vi"("error in (no error)"=w226, "Override Velosity Value"=w224, "Axis Select"=w225, "GECO Motion in"=w227) -> ("error out"=w222:errorcluster, "GECO Motion out"=w223:refnum<class "GECO Motion.lvclass">)  [unwired: 5 in, 1 out]
                  }
                }
              }
              frame 3 {
                n76 = Unbundle By Name(w229) -> ("二軸後退"=w228:bool)
                n77 = case shown="True" w228 {
                  tunnel: w234 -> [w244 w248]
                  tunnel: w233 -> [w243 w247]
                  tunnel: w232 -> [_ w256]
                  tunnel: [w235 w255] -> w231
                  tunnel: [w236 w254] -> w230
                  frame False {
                    w242 = u16 0 items=["Decelerate", "Halt"] ("Motion Stop Type")
                    n78 = call <vilib>:"Single Axis Move Stop.vi"("error in (no error)"=w243, "Motion Stop Type"=w242, "Axis Select"=Axis_Select."Axis 1", "GECO Motion in"=w244) -> ("error out"=w239:errorcluster, "Axis Select out"=w238:T4, "GECO Motion out"=w240:refnum<class "GECO Motion.lvclass">)  [unwired: 5 in]
                    n79 = call <vilib>:"Single Axis Load Velocity Override.vi"("error in (no error)"=w239, "Override Velosity Value"=0, "Axis Select"=w238, "GECO Motion in"=w240) -> ("error out"=w236:errorcluster, "GECO Motion out"=w235:refnum<class "GECO Motion.lvclass">)  [unwired: 5 in, 1 out]
                  }
                  frame True {
                    w246 = u16 0 items=["Decelerate", "Halt"] ("Motion Stop Type")
                    n80 = Multiply(x=-1, y=w256) -> (x*y=w253:i32)
                    n81 = call <vilib>:"Single Axis Move Stop.vi"("error in (no error)"=w247, "Motion Stop Type"=w246, "Axis Select"=Axis_Select."Axis 2", "GECO Motion in"=w248) -> ("error out"=w250:errorcluster, "Axis Select out"=w245:T4, "GECO Motion out"=w251:refnum<class "GECO Motion.lvclass">)  [unwired: 5 in]
                    n82 = call <vilib>:"Single Axis Move Start.vi"("error in (no error)"=w250, "Axis Select"=w245, "GECO Motion in"=w251) -> ("error out"=w258:errorcluster, "Axis Select out"=w257:T4, "GECO Motion out"=w259:refnum<class "GECO Motion.lvclass">)  [unwired: 6 in]
                    n83 = call <vilib>:"Single Axis Load Velocity Override.vi"("error in (no error)"=w258, "Override Velosity Value"=w253, "Axis Select"=w257, "GECO Motion in"=w259) -> ("error out"=w254:errorcluster, "GECO Motion out"=w255:refnum<class "GECO Motion.lvclass">)  [unwired: 5 in, 1 out]
                  }
                }
              }
              frame 4 {
                n84 = Unbundle By Name(w261) -> ("三軸前進"=w260:bool)
                n85 = case shown="False" w260 {
                  tunnel: w266 -> [w276 w282]
                  tunnel: w265 -> [w275 w281]
                  tunnel: w264 -> [_ w286]
                  tunnel: [w267 w285] -> w263
                  tunnel: [w268 w284] -> w262
                  frame False {
                    w274 = u16 0 items=["Decelerate", "Halt"] ("Motion Stop Type")
                    n86 = call <vilib>:"Single Axis Move Stop.vi"("error in (no error)"=w275, "Motion Stop Type"=w274, "Axis Select"=Axis_Select."Axis 1", "GECO Motion in"=w276) -> ("error out"=w271:errorcluster, "Axis Select out"=w270:T4, "GECO Motion out"=w272:refnum<class "GECO Motion.lvclass">)  [unwired: 5 in]
                    n87 = call <vilib>:"Single Axis Load Velocity Override.vi"("error in (no error)"=w271, "Override Velosity Value"=0, "Axis Select"=w270, "GECO Motion in"=w272) -> ("error out"=w268:errorcluster, "GECO Motion out"=w267:refnum<class "GECO Motion.lvclass">)  [unwired: 5 in, 1 out]
                  }
                  frame True {
                    w280 = u16 0 items=["Decelerate", "Halt"] ("Motion Stop Type")
                    n88 = call <vilib>:"Single Axis Move Stop.vi"("error in (no error)"=w281, "Motion Stop Type"=w280, "Axis Select"=Axis_Select."Axis 3", "GECO Motion in"=w282) -> ("error out"=w278:errorcluster, "Axis Select out"=w277:T4, "GECO Motion out"=w279:refnum<class "GECO Motion.lvclass">)  [unwired: 5 in]
                    n89 = call <vilib>:"Single Axis Move Start.vi"("error in (no error)"=w278, "Axis Select"=w277, "GECO Motion in"=w279) -> ("error out"=w288:errorcluster, "Axis Select out"=w287:T4, "GECO Motion out"=w289:refnum<class "GECO Motion.lvclass">)  [unwired: 6 in]
                    n90 = call <vilib>:"Single Axis Load Velocity Override.vi"("error in (no error)"=w288, "Override Velosity Value"=w286, "Axis Select"=w287, "GECO Motion in"=w289) -> ("error out"=w284:errorcluster, "GECO Motion out"=w285:refnum<class "GECO Motion.lvclass">)  [unwired: 5 in, 1 out]
                  }
                }
              }
              frame 5 {
                n91 = Unbundle By Name(w291) -> ("三軸後退"=w290:bool)
                n92 = case shown="False" w290 {
                  tunnel: w296 -> [w306 w310]
                  tunnel: w295 -> [w305 w309]
                  tunnel: w294 -> [_ w318]
                  tunnel: [w297 w317] -> w293
                  tunnel: [w298 w316] -> w292
                  frame False {
                    w304 = u16 0 items=["Decelerate", "Halt"] ("Motion Stop Type")
                    n93 = call <vilib>:"Single Axis Move Stop.vi"("error in (no error)"=w305, "Motion Stop Type"=w304, "Axis Select"=Axis_Select."Axis 1", "GECO Motion in"=w306) -> ("error out"=w301:errorcluster, "Axis Select out"=w300:T4, "GECO Motion out"=w302:refnum<class "GECO Motion.lvclass">)  [unwired: 5 in]
                    n94 = call <vilib>:"Single Axis Load Velocity Override.vi"("error in (no error)"=w301, "Override Velosity Value"=0, "Axis Select"=w300, "GECO Motion in"=w302) -> ("error out"=w298:errorcluster, "GECO Motion out"=w297:refnum<class "GECO Motion.lvclass">)  [unwired: 5 in, 1 out]
                  }
                  frame True {
                    w308 = u16 0 items=["Decelerate", "Halt"] ("Motion Stop Type")
                    n95 = Multiply(x=-1, y=w318) -> (x*y=w315:i32)
                    n96 = call <vilib>:"Single Axis Move Stop.vi"("error in (no error)"=w309, "Motion Stop Type"=w308, "Axis Select"=Axis_Select."Axis 3", "GECO Motion in"=w310) -> ("error out"=w312:errorcluster, "Axis Select out"=w307:T4, "GECO Motion out"=w313:refnum<class "GECO Motion.lvclass">)  [unwired: 5 in]
                    n97 = call <vilib>:"Single Axis Move Start.vi"("error in (no error)"=w312, "Axis Select"=w307, "GECO Motion in"=w313) -> ("error out"=w320:errorcluster, "Axis Select out"=w319:T4, "GECO Motion out"=w321:refnum<class "GECO Motion.lvclass">)  [unwired: 6 in]
                    n98 = call <vilib>:"Single Axis Load Velocity Override.vi"("error in (no error)"=w320, "Override Velosity Value"=w315, "Axis Select"=w319, "GECO Motion in"=w321) -> ("error out"=w316:errorcluster, "GECO Motion out"=w317:refnum<class "GECO Motion.lvclass">)  [unwired: 5 in, 1 out]
                  }
                }
              }
              frame 6 {
                n99 = Unbundle By Name(w323) -> ("三軸同進"=w322:bool)
                n100 = case shown="False" w322 {
                  tunnel: w328 -> [w332 w350]
                  tunnel: w327 -> [w333 w349]
                  tunnel: w326 -> [_ w345]
                  tunnel: [w330 w358] -> w325
                  tunnel: [w329 w357] -> w324
                  frame False {
                    w331 = T4[] [enum."Axis 1", enum."Axis 2", enum."Axis 3"] items=["Axis 1", "Axis 2", "Axis 3", "Axis 4"] ("Start Axes Select")
                    n101 = for {
                      tunnel: w333 -> [w342]
                      tunnel: w332 -> [w341]
                      tunnel: w331 -> [w340] mode=indexing
                      tunnel: [w335] -> w330
                      tunnel: [w336] -> w329
                      w343 = u16 0 items=["Decelerate", "Halt"] ("Motion Stop Type")
                      n102 = call <vilib>:"Single Axis Move Stop.vi"("error in (no error)"=w342, "Motion Stop Type"=w343, "Axis Select"=w340, "GECO Motion in"=w341) -> ("error out"=w338:errorcluster, "Axis Select out"=w337:T4, "GECO Motion out"=w339:refnum<class "GECO Motion.lvclass">)  [unwired: 5 in]
                      n103 = call <vilib>:"Single Axis Load Velocity Override.vi"("error in (no error)"=w338, "Override Velosity Value"=0, "Axis Select"=w337, "GECO Motion in"=w339) -> ("error out"=w336:errorcluster, "GECO Motion out"=w335:refnum<class "GECO Motion.lvclass">)  [unwired: 5 in, 1 out]
                    }
                  }
                  frame True {
                    w346 = T4[] [enum."Axis 1", enum."Axis 2", enum."Axis 3"] items=["Axis 1", "Axis 2", "Axis 3", "Axis 4"] ("Start Axes Select")
                    n104 = call <vilib>:"Single Axis Load Velocity Override.vi"("error in (no error)"=w349, "Override Velosity Value"=w345, "Axis Select"=Axis_Select."Axis 1", "GECO Motion in"=w350) -> ("error out"=w355:errorcluster, "GECO Motion out"=w356:refnum<class "GECO Motion.lvclass">)  [unwired: 5 in, 1 out]
                    n105 = call <vilib>:"Single Axis Load Velocity Override.vi"("error in (no error)"=w355, "Override Velosity Value"=w345, "Axis Select"=Axis_Select."Axis 2", "GECO Motion in"=w356) -> ("error out"=w353:errorcluster, "GECO Motion out"=w354:refnum<class "GECO Motion.lvclass">)  [unwired: 5 in, 1 out]
                    n106 = call <vilib>:"Single Axis Load Velocity Override.vi"("error in (no error)"=w353, "Override Velosity Value"=w345, "Axis Select"=Axis_Select."Axis 3", "GECO Motion in"=w354) -> ("error out"=w351:errorcluster, "GECO Motion out"=w352:refnum<class "GECO Motion.lvclass">)  [unwired: 5 in, 1 out]
                    n107 = call <vilib>:"MultiAxes Sync Move Start.vi"("error in (no error)"=w351, "Start Axes Select"=w346, "GECO Motion in"=w352) -> ("error out"=w357:errorcluster, "GECO Motion out"=w358:refnum<class "GECO Motion.lvclass">)  [unwired: 7 in]
                  }
                }
              }
              frame 7 {
                n108 = Unbundle By Name(w360) -> ("三軸同退"=w359:bool)
                n109 = case shown="False" w359 {
                  tunnel: w365 -> [w369 w389]
                  tunnel: w364 -> [w370 w388]
                  tunnel: w363 -> [_ w382]
                  tunnel: [w367 w397] -> w362
                  tunnel: [w366 w396] -> w361
                  frame False {
                    w368 = T4[] [enum."Axis 1", enum."Axis 2", enum."Axis 3"] items=["Axis 1", "Axis 2", "Axis 3", "Axis 4"] ("Start Axes Select")
                    n110 = for {
                      tunnel: w370 -> [w379]
                      tunnel: w369 -> [w378]
                      tunnel: w368 -> [w377] mode=indexing
                      tunnel: [w372] -> w367
                      tunnel: [w373] -> w366
                      w380 = u16 0 items=["Decelerate", "Halt"] ("Motion Stop Type")
                      n111 = call <vilib>:"Single Axis Move Stop.vi"("error in (no error)"=w379, "Motion Stop Type"=w380, "Axis Select"=w377, "GECO Motion in"=w378) -> ("error out"=w375:errorcluster, "Axis Select out"=w374:T4, "GECO Motion out"=w376:refnum<class "GECO Motion.lvclass">)  [unwired: 5 in]
                      n112 = call <vilib>:"Single Axis Load Velocity Override.vi"("error in (no error)"=w375, "Override Velosity Value"=0, "Axis Select"=w374, "GECO Motion in"=w376) -> ("error out"=w373:errorcluster, "GECO Motion out"=w372:refnum<class "GECO Motion.lvclass">)  [unwired: 5 in, 1 out]
                    }
                  }
                  frame True {
                    w385 = T4[] [enum."Axis 1", enum."Axis 2", enum."Axis 3"] items=["Axis 1", "Axis 2", "Axis 3", "Axis 4"] ("Start Axes Select")
                    n113 = Multiply(x=w382, y=-1) -> (x*y=w383:i32)
                    n114 = call <vilib>:"Single Axis Load Velocity Override.vi"("error in (no error)"=w388, "Override Velosity Value"=w383, "Axis Select"=Axis_Select."Axis 1", "GECO Motion in"=w389) -> ("error out"=w394:errorcluster, "GECO Motion out"=w395:refnum<class "GECO Motion.lvclass">)  [unwired: 5 in, 1 out]
                    n115 = call <vilib>:"Single Axis Load Velocity Override.vi"("error in (no error)"=w394, "Override Velosity Value"=w383, "Axis Select"=Axis_Select."Axis 2", "GECO Motion in"=w395) -> ("error out"=w392:errorcluster, "GECO Motion out"=w393:refnum<class "GECO Motion.lvclass">)  [unwired: 5 in, 1 out]
                    n116 = call <vilib>:"Single Axis Load Velocity Override.vi"("error in (no error)"=w392, "Override Velosity Value"=w383, "Axis Select"=Axis_Select."Axis 3", "GECO Motion in"=w393) -> ("error out"=w390:errorcluster, "GECO Motion out"=w391:refnum<class "GECO Motion.lvclass">)  [unwired: 5 in, 1 out]
                    n117 = call <vilib>:"MultiAxes Sync Move Start.vi"("error in (no error)"=w390, "Start Axes Select"=w385, "GECO Motion in"=w391) -> ("error out"=w396:errorcluster, "GECO Motion out"=w397:refnum<class "GECO Motion.lvclass">)  [unwired: 7 in]
                  }
                }
              }
            }
            n118 = Bundle By Name(cluster=w112, "GECO Motion out"=w113) -> (w118:T3)
          }
          frame "ZABMove" {
            w399 = T4[] [enum."Axis 1", enum."Axis 2", enum."Axis 3"] items=["Axis 1", "Axis 2", "Axis 3", "Axis 4"] ("Start Axes Select")
            n119 = Unbundle By Name(w410) -> ("PIDSetting.Move Setting"=w411:T9, "GECO Motion out"=w400:refnum<class "GECO Motion.lvclass">)
            n120 = call <vilib>:"MultiAxes Sync Move Start.vi"("error in (no error)"=w401, "Start Axes Select"=w399, "GECO Motion in"=w400) -> ("error out"=w402:errorcluster, "GECO Motion out"=w403:refnum<class "GECO Motion.lvclass">)  [unwired: 7 in]
            n121 = case shown="1" w411 {
              selector: w411 -> [_ w426 w533 _ _]
              tunnel: w410 -> [_ w448 w530 w536 w539]
              tunnel: w402 -> [w416 w457 w532 w535 w538]
              tunnel: [w415 w423 w484 w535 w538] -> w409
              tunnel: [w414 w427 w485 w534 w537] -> w407
              tunnel: [_ _ w471 _ _] -> w406
              tunnel: [_ _ w470 _ _] -> w405
              tunnel: [_ _ w469 _ _] -> w404
              tunnel: w403 -> [w412 _ w531 _ _]
              tunnel: [_ _ w472 _ _] -> w398
              frame Default {
                w413 = T4[] [enum."Axis 1", enum."Axis 2", enum."Axis 3", enum."Axis 4"] items=["Axis 1", "Axis 2", "Axis 3", "Axis 4"]
                n122 = for {
                  tunnel: w416 -> [w419]
                  tunnel: [w417] -> w415
                  tunnel: [w418] -> w414
                  tunnel: w413 -> [w421] mode=indexing
                  tunnel: w412 -> [w422]
                  w420 = u16 0 items=["Decelerate", "Halt"] ("Motion Stop Type")
                  n123 = call <vilib>:"Single Axis Move Stop.vi"("error in (no error)"=w419, "Motion Stop Type"=w420, "Axis Select"=w421, "GECO Motion in"=w422) -> ("error out"=w417:errorcluster, "GECO Motion out"=w418:refnum<class "GECO Motion.lvclass">)  [unwired: 5 in, 1 out]
                }
              }
              frame 0 {
                w436 = T4[] [enum."Axis 1", enum."Axis 2", enum."Axis 3"] items=["Axis 1", "Axis 2", "Axis 3", "Axis 4"] ("Start Axes Select")
                # "輸入Z、A、B"
                n124 = Unbundle By Name(w448) -> ("PIDSetting.Z"=w454:i32, "PIDSetting.A"=w453:i32, "PIDSetting.B"=w452:i32, "PIDSetting.Axis Length"=w462:dbl, "PIDSetting.Axis Pulse"=w458:dbl, "GECO Motion out"=w456:refnum<class "GECO Motion.lvclass">)
                n125 = Unbundle By Name(w448) -> ("ServoSetting.Singel Axis Move Paramters.Velocity (10000)"=w431:i32)
                n126 = call "綜合圓軌跡子VI.vi"("Ring"=w426, "移動z"=w454, "al"=w453, "be"=w452) -> ("Z"=w428:dbl, "A"=w429:dbl, "B"=w430:dbl)  [unwired: 2 in]
                n127 = call "推導公式.vi"("be"=w430, "al"=w429, "移動z"=w428) -> ("L3"=w463:dbl, "L2"=w464:dbl, "L1"=w465:dbl)
                n128 = Subtract(x=w465, y=w462) -> (x-y=w461:dbl)
                n129 = Subtract(x=w464, y=w462) -> (x-y=w460:dbl)
                n130 = Subtract(x=w463, y=w462) -> (x-y=w459:dbl)
                n131 = Multiply(x=w461, y=w458) -> (x*y=w424:dbl)
                n132 = Multiply(x=w460, y=w458) -> (x*y=w433:dbl)
                n133 = Multiply(x=w459, y=w458) -> (x*y=w425:dbl)
                n134 = call <vilib>:"Single Axis Load Velocity Override.vi"("error in (no error)"=w457, "Override Velosity Value"=w431, "Axis Select"=Axis_Select."Axis 1" ("Single Axis Select"), "GECO Motion in"=w456) -> ("error out"=w450:errorcluster, "Axis Select out"=w449:T4, "GECO Motion out"=w451:refnum<class "GECO Motion.lvclass">)  [unwired: 5 in]
                n135 = call <vilib>:"Single Axis Load Position Override.vi"("error in (no error)"=w450, "Override Target Position Value"=w425, "Axis Select"=w449, "GECO Motion in"=w451) -> ("error out"=w446:errorcluster, "GECO Motion out"=w447:refnum<class "GECO Motion.lvclass">)  [unwired: 5 in, 1 out]
                n136 = call <vilib>:"Single Axis Load Velocity Override.vi"("error in (no error)"=w446, "Override Velosity Value"=w431, "Axis Select"=Axis_Select."Axis 2" ("Single Axis Select"), "GECO Motion in"=w447) -> ("error out"=w443:errorcluster, "Axis Select out"=w442:T4, "GECO Motion out"=w444:refnum<class "GECO Motion.lvclass">)  [unwired: 5 in]
                n137 = call <vilib>:"Single Axis Load Position Override.vi"("error in (no error)"=w443, "Override Target Position Value"=w433, "Axis Select"=w442, "GECO Motion in"=w444) -> ("error out"=w437:errorcluster, "GECO Motion out"=w438:refnum<class "GECO Motion.lvclass">)  [unwired: 5 in, 1 out]
                n138 = call <vilib>:"Single Axis Load Velocity Override.vi"("error in (no error)"=w437, "Override Velosity Value"=w431, "Axis Select"=Axis_Select."Axis 3" ("Single Axis Select"), "GECO Motion in"=w438) -> ("error out"=w440:errorcluster, "Axis Select out"=w439:T4, "GECO Motion out"=w441:refnum<class "GECO Motion.lvclass">)  [unwired: 5 in]
                n139 = call <vilib>:"Single Axis Load Position Override.vi"("error in (no error)"=w440, "Override Target Position Value"=w424, "Axis Select"=w439, "GECO Motion in"=w441) -> ("error out"=w434:errorcluster, "GECO Motion out"=w435:refnum<class "GECO Motion.lvclass">)  [unwired: 5 in, 1 out]
                n140 = call <vilib>:"MultiAxes Sync Move Start.vi"("error in (no error)"=w434, "Start Axes Select"=w436, "GECO Motion in"=w435) -> ("error out"=w423:errorcluster, "GECO Motion out"=w427:refnum<class "GECO Motion.lvclass">)  [unwired: 7 in]
              }
              frame 1 {
                w529 = cluster{"output high":dbl, "output low":dbl} {"output high"=200000.0, "output low"=-500000.0} ("PID Def Output range")
                w497 = Axis_Select."Axis 3" ("Single Axis Select")
                w498 = Axis_Select."Axis 2" ("Single Axis Select")
                w496 = Axis_Select."Axis 1" ("Single Axis Select")
                # "PID取樣時間"
                # "Stm32 Delay Time"
                # "圓軌跡"
                n141 = Unbundle By Name(w530) -> ("PIDSetting.Axis Length"=w505:dbl, "PIDSetting.Axis Pulse"=w519:dbl)
                n142 = feedback #1() -> (w476:i32)
                n143 = Increment(x=w476) -> (x+1=w477:i32)
                n144 = feedback-in #1(w477) -> ()
                n145 = call <vilib>:"Read Encoder Position.vi"("error in (no error)"=w532, "Axis Select"=w496, "GECO Motion in"=w531) -> ("error out"=w503:errorcluster, "GECO Motion out"=w504:refnum<class "GECO Motion.lvclass">, "Encoder Position"=w483:i32, "Logical Position"=w495:i32)  [unwired: 4 in, 1 out]
                n146 = call <vilib>:"Read Encoder Position.vi"("error in (no error)"=w503, "Axis Select"=w498, "GECO Motion in"=w504) -> ("error out"=w501:errorcluster, "GECO Motion out"=w502:refnum<class "GECO Motion.lvclass">, "Encoder Position"=w482:i32, "Logical Position"=w494:i32)  [unwired: 4 in, 1 out]
                n147 = Bundle("Encoder Position"=w483, "Logical Position"=w495) -> (w471:T1)  [unwired: 1 in]
                n148 = call <vilib>:"Read Encoder Position.vi"("error in (no error)"=w501, "Axis Select"=w497, "GECO Motion in"=w502) -> ("error out"=w499:errorcluster, "GECO Motion out"=w500:refnum<class "GECO Motion.lvclass">, "Encoder Position"=w481:i32, "Logical Position"=w493:i32)  [unwired: 4 in, 1 out]
                n149 = call "綜合圓軌跡子VI.vi"("Ring"=w533, "I時間"=w476) -> ("Z"=w526:dbl, "A"=w475:dbl, "B"=w474:dbl)  [unwired: 4 in]
                n150 = property on="Axis 1" class="Clust (strict)"("Value"=w471) -> ()  [unwired: 2 in, 2 out]
                n151 = call "推導公式.vi"("be"=w474, "al"=w475, "移動z"=w526) -> ("L3"=w520:dbl, "L2"=w521:dbl, "L1"=w522:dbl)
                n152 = shared-variable "My Computer\\PC_Variables.lvlib\\PID gains"() -> (w468:T23)  [unwired: 1 in, 1 out]
                n153 = shared-variable "My Computer\\PC_Variables.lvlib\\PID gains 2"() -> (w467:T23)  [unwired: 1 in, 1 out]
                n154 = shared-variable "My Computer\\PC_Variables.lvlib\\PID gains 3"() -> (w466:T23)  [unwired: 1 in, 1 out]
                n155 = Bundle("Encoder Position"=w482, "Logical Position"=w494) -> (w470:T1)  [unwired: 1 in]
                n156 = Subtract(x=w522, y=w505) -> (x-y=w525:dbl)
                n157 = Subtract(x=w521, y=w505) -> (x-y=w524:dbl)
                n158 = Subtract(x=w520, y=w505) -> (x-y=w523:dbl)
                n159 = property on="Axis 2" class="Clust (strict)"("Value"=w470) -> ()  [unwired: 2 in, 2 out]
                n160 = feedback #2() -> (w480:i32)
                n161 = feedback-in #2(w483) -> ()
                n162 = feedback #3() -> (w479:i32)
                n163 = feedback-in #3(w482) -> ()
                n164 = feedback #4() -> (w478:i32)
                n165 = feedback-in #4(w481) -> ()
                n166 = Multiply ("L1 pulse")(x=w525, y=w519) -> (x*y=w491:dbl)
                n167 = Multiply ("L2 pulse")(x=w524, y=w519) -> (x*y=w490:dbl)
                n168 = Multiply ("L3 pulse")(x=w523, y=w519) -> (x*y=w489:dbl)
                n169 = Divide(x=25.0, y=1000.0) -> (x/y=w518:dbl)
                n170 = Bundle("Encoder Position"=w481, "Logical Position"=w493) -> (w469:T1)  [unwired: 1 in]
                n171 = property on="Axis 3" class="Clust (strict)"("Value"=w469) -> ()  [unwired: 2 in, 2 out]
                n172 = call-poly <vilib>:"PID.vi"("output range"=w529, "dt (s)"=w518, "PID gains"=w468, "process variable"=w480, "setpoint"=w489) -> ("output"=w488:dbl)  [unwired: 5 in, 1 out]
                n173 = call-poly <vilib>:"PID.vi"("output range"=w529, "dt (s)"=w518, "PID gains"=w467, "process variable"=w479, "setpoint"=w490) -> ("output"=w487:dbl)  [unwired: 5 in, 1 out]
                n174 = call-poly <vilib>:"PID.vi"("output range"=w529, "dt (s)"=w518, "PID gains"=w466, "process variable"=w478, "setpoint"=w491) -> ("output"=w486:dbl)  [unwired: 5 in, 1 out]
                n175 = call <vilib>:"Single Axis Load Velocity Override.vi"("error in (no error)"=w499, "Override Velosity Value"=w488, "Axis Select"=w496, "GECO Motion in"=w500) -> ("error out"=w516:errorcluster, "Axis Select out"=w508:T4, "GECO Motion out"=w517:refnum<class "GECO Motion.lvclass">)  [unwired: 5 in]
                n176 = call <vilib>:"Single Axis Load Position Override.vi"("error in (no error)"=w516, "Axis Select"=w508, "GECO Motion in"=w517) -> ("error out"=w514:errorcluster, "GECO Motion out"=w515:refnum<class "GECO Motion.lvclass">)  [unwired: 6 in, 1 out]
                n177 = shared-variable "My Computer\\PC_Variables.lvlib\\Axis 1 Position"(w471) -> ()  [unwired: 1 in, 1 out]
                n178 = call <vilib>:"Single Axis Load Velocity Override.vi"("error in (no error)"=w514, "Override Velosity Value"=w487, "Axis Select"=w498, "GECO Motion in"=w515) -> ("error out"=w492:errorcluster, "Axis Select out"=w507:T4, "GECO Motion out"=w513:refnum<class "GECO Motion.lvclass">)  [unwired: 5 in]
                n179 = call <vilib>:"Single Axis Load Position Override.vi"("error in (no error)"=w492, "Axis Select"=w507, "GECO Motion in"=w513) -> ("error out"=w511:errorcluster, "GECO Motion out"=w512:refnum<class "GECO Motion.lvclass">)  [unwired: 6 in, 1 out]
                n180 = call <vilib>:"Single Axis Load Velocity Override.vi"("error in (no error)"=w511, "Override Velosity Value"=w486, "Axis Select"=w497, "GECO Motion in"=w512) -> ("error out"=w509:errorcluster, "Axis Select out"=w506:T4, "GECO Motion out"=w510:refnum<class "GECO Motion.lvclass">)  [unwired: 5 in]
                n181 = shared-variable "My Computer\\PC_Variables.lvlib\\Axis 2 Position"(w470) -> ()  [unwired: 1 in, 1 out]
                n182 = call <vilib>:"Single Axis Load Position Override.vi"("error in (no error)"=w509, "Axis Select"=w506, "GECO Motion in"=w510) -> ("error out"=w484:errorcluster, "GECO Motion out"=w485:refnum<class "GECO Motion.lvclass">)  [unwired: 6 in, 1 out]
                n183 = shared-variable "My Computer\\PC_Variables.lvlib\\Axis 3 Position"(w469) -> ()  [unwired: 1 in, 1 out]
                n184 = Bundle By Name(cluster=cluster{"A":dbl, "B":dbl} {"A"=0.0, "B"=0.0} ("理想角度"), "A"=w475, "B"=w474) -> (w472:cluster{"A":dbl, "B":dbl})
              }
              frame 2 {
                # "Á³±Û­y¸ñ"
                n185 = Unbundle By Name(w536) -> ("GECO Motion out"=w534:refnum<class "GECO Motion.lvclass">)
              }
              frame 3 {
                # "Z上下"
                n186 = Unbundle By Name(w539) -> ("GECO Motion out"=w537:refnum<class "GECO Motion.lvclass">)
              }
            }
            n187 = Bundle By Name(cluster=w410, "GECO Motion out"=w407, "Axis 1 Position"=w406, "Axis 2 Position"=w405, "Axis 3 Position"=w404, "理想角度"=w398) -> (w408:T3)
          }
          frame "AlarmReset" {
            w546 = T4[] [enum."Axis 1", enum."Axis 2", enum."Axis 3", enum."Axis 4"] items=["Axis 1", "Axis 2", "Axis 3", "Axis 4"]
            n188 = Unbundle By Name(w545) -> ("GECO Motion out"=w543:refnum<class "GECO Motion.lvclass">)
            n189 = for {
              tunnel: [w555] -> w541
              tunnel: [w554] -> w540
              tunnel: w546 -> [w549] mode=indexing
              tunnel: w544 -> [w551]
              tunnel: w543 -> [w550]
              w547 = u16 0 items=["Decelerate", "Halt"] ("Motion Stop Type")
              n190 = call <vilib>:"Single Axis Move Stop.vi"("error in (no error)"=w551, "Motion Stop Type"=w547, "Axis Select"=w549, "GECO Motion in"=w550) -> ("error out"=w552:errorcluster, "Axis Select out"=w548:T4, "GECO Motion out"=w553:refnum<class "GECO Motion.lvclass">)  [unwired: 5 in]
              n191 = call <vilib>:"Alarm Reset.vi"("error in (no error)"=w552, "Axis Select"=w548, "GECO Motion in"=w553) -> ("error out"=w554:errorcluster, "GECO Motion out"=w555:refnum<class "GECO Motion.lvclass">)  [unwired: 6 in, 1 out]
            }
            n192 = Bundle By Name(cluster=w545, "GECO Motion out"=w541) -> (w542:T3)
          }
          frame "EncoderReset" {
            w562 = T4[] [enum."Axis 1", enum."Axis 2", enum."Axis 3", enum."Axis 4"] items=["Axis 1", "Axis 2", "Axis 3", "Axis 4"]
            n193 = Unbundle By Name(w561) -> ("GECO Motion out"=w559:refnum<class "GECO Motion.lvclass">)
            n194 = for {
              tunnel: [w571] -> w557
              tunnel: [w570] -> w556
              tunnel: w562 -> [w569] mode=indexing
              tunnel: w560 -> [w566]
              tunnel: w559 -> [w565]
              w563 = u16 0 items=["Decelerate", "Halt"] ("Motion Stop Type")
              n195 = call <vilib>:"Single Axis Move Stop.vi"("error in (no error)"=w566, "Motion Stop Type"=w563, "Axis Select"=w569, "GECO Motion in"=w565) -> ("error out"=w567:errorcluster, "Axis Select out"=w564:T4, "GECO Motion out"=w568:refnum<class "GECO Motion.lvclass">)  [unwired: 5 in]
              n196 = call <vilib>:"Reset Encoder Position.vi"("error in (no error)"=w567, "Axis Select"=w564, "GECO Motion in"=w568) -> ("error out"=w570:errorcluster, "GECO Motion out"=w571:refnum<class "GECO Motion.lvclass">)  [unwired: 6 in, 1 out]
            }
            n197 = Bundle By Name(cluster=w561, "GECO Motion out"=w557) -> (w558:T3)
          }
          frame "LinkBoard" {
            n198 = Unbundle By Name(w592) -> ("resource name"=w582:tag, "TCP slave port"=w590:u16, "ServoSetting.Motion Controller Slot"=w583:T7)
            n199 = Format Date/Time String(time format string (%c)="%Y %m %d %H %M ") -> (date/time string=w579:string)  [unwired: 2 in]
            n200 = Concatenate Strings(w579, "Ideal Angle.txt" ("element")) -> (w578:string)
            n201 = Build Path(base path=path "u:/data", name or relative path=w578) -> (appended path=w580:path)
            n202 = Open/Create/Replace File(file path (use dialog)=w580, error in=w574, operation (0:open)=T19."replace or create") -> (refnum out=w572:refnum<file>, error out=w575:errorcluster)  [unwired: 3 in, 1 out]
            n203 = call-poly <vilib>:"Create Modbus Instance.vi"("error in"=w575, "port (502)"=w590) -> ("error out"=w589:errorcluster, "TCP slave instance"=w584:refnum<class "Modbus Slave.lvclass">)  [unwired: 8 in]
            n204 = call-poly <vilib>:"InitializeRT.vi"("error in (no error)"=w589, "resource name"=w582) -> ("error out"=w588:errorcluster, "GECO_Driver out"=w585:refnum<class "GECO_Driver.lvclass">)  [unwired: 8 in]
            n205 = call <vilib>:"Initialize Motion Controller.vi"("error in (no error)"=w588, "Slot"=w583, "GECO_Driver in"=w585) -> ("error out"=w586:errorcluster, "Motion reference out"=w587:refnum<class "GECO Motion.lvclass">)  [unwired: 7 in]
            n206 = Bundle By Name(cluster=w592, "Modbus COM"=w584, "GECO_Driver out"=w585, "GECO Motion out"=w587, "Save Path"=w572) -> (w591:T3)
          }
          frame "PanelUpdate" {
            n207 = Unbundle By Name(w615) -> ("GECO Motion out"=w614:refnum<class "GECO Motion.lvclass">)
            n208 = call <vilib>:"Read Encoder Position.vi"("error in (no error)"=w617, "Axis Select"=Axis_Select."Axis 1", "GECO Motion in"=w614) -> ("error out"=w610:errorcluster, "GECO Motion out"=w611:refnum<class "GECO Motion.lvclass">, "Encoder Position"=w603:i32, "Logical Position"=w604:i32)  [unwired: 4 in, 1 out]
            n209 = Bundle(cluster=T20 {"Logical Position"=0, "Encoder Position"=0} ("input cluster"), "Logical Position"=w604, "Encoder Position"=w603) -> (w595:T20)
            "Axis 1" <- w595
            n210 = shared-variable "My Computer\\PC_Variables.lvlib\\Axis 1 Position"(w595) -> ()  [unwired: 1 in, 1 out]
            n211 = call <vilib>:"Read Encoder Position.vi"("error in (no error)"=w610, "Axis Select"=Axis_Select."Axis 2", "GECO Motion in"=w611) -> ("error out"=w608:errorcluster, "GECO Motion out"=w609:refnum<class "GECO Motion.lvclass">, "Encoder Position"=w596:i32, "Logical Position"=w597:i32)  [unwired: 4 in, 1 out]
            n212 = Bundle(cluster=T20 {"Logical Position"=0, "Encoder Position"=0} ("input cluster"), "Logical Position"=w597, "Encoder Position"=w596) -> (w594:T20)
            "Axis 2" <- w594
            n213 = shared-variable "My Computer\\PC_Variables.lvlib\\Axis 2 Position"(w594) -> ()  [unwired: 1 in, 1 out]
            n214 = call <vilib>:"Read Encoder Position.vi"("error in (no error)"=w608, "Axis Select"=Axis_Select."Axis 3", "GECO Motion in"=w609) -> ("error out"=w616:errorcluster, "GECO Motion out"=w612:refnum<class "GECO Motion.lvclass">, "Encoder Position"=w598:i32, "Logical Position"=w599:i32)  [unwired: 4 in, 1 out]
            n215 = Bundle(cluster=T20 {"Logical Position"=0, "Encoder Position"=0} ("input cluster"), "Logical Position"=w599, "Encoder Position"=w598) -> (w593:T20)
            "Axis 3" <- w593
            n216 = shared-variable "My Computer\\PC_Variables.lvlib\\Axis 3 Position"(w593) -> ()  [unwired: 1 in, 1 out]
            n217 = Bundle By Name(cluster=w615, "GECO Motion out"=w612, "Axis 1 Position"=w595, "Axis 2 Position"=w594, "Axis 3 Position"=w593) -> (w613:T3)
          }
          frame "CloseBoard" {
            w618 = T4[] [enum."Axis 1", enum."Axis 2", enum."Axis 3", enum."Axis 4"] items=["Axis 1", "Axis 2", "Axis 3", "Axis 4"]
            n218 = Unbundle By Name(w624) -> ("GECO_Driver out"=w620:refnum<class "GECO_Driver.lvclass">, "GECO Motion out"=w619:refnum<class "GECO Motion.lvclass">)
            n219 = for {
              tunnel: [w629] -> w621
              tunnel: w619 -> [w628]
              tunnel: w622 -> [w627]
              tunnel: w618 -> [w625] mode=indexing
              n220 = call <vilib>:"Servo On.vi"("error in (no error)"=w627, "Servo On"=FALSE, "Axis Select"=w625, "GECO Motion in"=w628) -> ("error out"=w632:errorcluster, "Axis Select out"=w631:T4, "GECO Motion out"=w630:refnum<class "GECO Motion.lvclass">)  [unwired: 5 in]
              n221 = call <vilib>:"Single Axis Move Stop.vi"("error in (no error)"=w632, "Axis Select"=w631, "GECO Motion in"=w630) -> ("error out"=w629:errorcluster)  [unwired: 6 in, 2 out]
            }
            n222 = call <vilib>:"Close.vi"("error in (no error)"=w621, "GECO_Driver in"=w620) -> ("error out"=w623:errorcluster)  [unwired: 9 in]
          }
        }
        "error out" <- w25
        n223 = shared-variable "NI-sbRIO9606-01F1BAB2\\RT_Variables.lvlib\\error out"(w25) -> ()  [unwired: 1 in, 1 out]
        n224 = Unbundle By Name(w25) -> ("status"=w26:bool)
      }
      frame Error {
      }
    }
    n225 = Tick Count (ms)() -> (millisecond timer value=w18:u32)
    n226 = Unbundle By Name(w16) -> ("理想角度"=w15:cluster{"A":dbl, "B":dbl})
    n227 = Subtract(x=w18, y=w17) -> (x-y=w14:u32)
    "Program Period" <- w14
    n228 = shared-variable "NI-sbRIO9606-01F1BAB2\\RT_Variables.lvlib\\Program Period"(w14) -> ()  [unwired: 1 in, 1 out]
    n229 = node-c288() -> ()  [unwired: 1 in, 1 out]
  }
  n230 = node-c288(w1) -> ()  [unwired: 1 out]
  n231 = Unbundle By Name(w5) -> ("Save Path"=w4:refnum<file>)
  n232 = for {
    tunnel: [w645] -> w3 mode=indexing
    tunnel: w7 -> [w644] mode=indexing
    tunnel: w6 -> [w641] mode=indexing
    n233 = Unbundle(w644) -> ("A"=w643:dbl, "B"=w642:dbl)
    n234 = Format Into String(w643) -> (resulting string=w638:string)  [unwired: 3 in, 1 out]
    n235 = Format Into String(w642) -> (resulting string=w636:string)  [unwired: 3 in, 1 out]
    n236 = Format Into String(w641) -> (resulting string=w640:string)  [unwired: 3 in, 1 out]
    n237 = Insert Into Array(array=string[] ["Program Period(ms)："], new element #1=w640, new element #2="A：", new element #3=w638, new element #4="B：", new element #5=w636) -> (w645:string[])  [unwired: 1 in]
  }
  n238 = for {
    tunnel: w3 -> [w649] mode=indexing
    shift-right: [w647] -> _
    shift-left: w4 -> [w651]
    shift-right: [w648] -> _
    shift-left: _ -> [w650]
    n239 = Array To Spreadsheet String(delimiter (Tab)="\t", array=w649, 3:"%f" ("format string")) -> (spreadsheet string=w652:string)
    n240 = Write to Text File(file (use dialog)=w651, text=w652, error in=w650) -> (refnum out=w647:refnum<file>, error out=w648:errorcluster)  [unwired: 1 in, 1 out]
  }
